vi "Quantum Composers 9000 Series Recall-Save Configuration.vi"() -> ()   [LabVIEW 2012]
doc: "This VI is an example of how to use subVIs from the QC 9000 series driver to programmatically recall/save a configuration from/to the unit's non-volatile memory.\n\n\nNotes:\n1) The pulse generator keypad is returned to \"Local\" mode when this VI terminates in order to restore manual control to the user.\n2) VISA Version 3.3 or higher must be installed to use this instrument driver."
uses:
  Support/Channel Parameters.ctl
  Support/System Parameters.ctl
  Quantum Composers 9000 Series.lvlib
panel:
  in  "Recall/Save (F:Read)":bool
  in  "Memory  (1)":i32=1
  in  "System Parameters":T1={"Sys Period"=0.1, "Sys Mode"=enum."Normal", "Sys Burst #"=10, "Sys DC On"=10, "Sys DC Off"=10, "Sys State"=TRUE, "Sys Gate"=TRUE, "Sys Trig Edge"=TRUE, "Sys Ext Mode"=enum."Disabled", "Sys Trig Lev"=2.5, "Sys Gate Lev "=2.5, "Sys Gate Mode"=enum."Disabled"} {"Sys Gate Lev" format="%.4p"; "Sys Trig Lev" format="%.4p"; "Sys Period" format="%.6p"}
  in  "VISA resource":refnum<visa-resource-name>="GPIB0::7::INSTR"
  in  "Channel Parameters":T2[](array[typedef]) {"Chan Sync Source" items=["System (To)", "Channel A", "Channel B", "Channel C", "Channel D", "Channel E", "Channel F", "Channel G", "Channel H"]; "Chan Width" format="%.3p"; "Chan Delay" format="%.3p"; "Chan Lev Adjust" format="%.3p"; "Channel" items=["Channel A"=1, "Channel B"=2, "Channel C"=3, "Channel D"=4, "Channel E"=5, "Channel F"=6, "Channel G"=7, "Channel H"=8]}
  # "9000 Series\nPulse Generator\nExample Program"
  # "Notes:\n1.  The channel parameters \"Burst #\", \"DC On\", \"DC Off\", and \"Adjustable\" are only updated when operating in the corresponding mode.\n2.  The system parameters  \"Burst #\", \"DC On\", \"DC Off\", and \"Trig Level\"` are only updated when operating in the corresponding mode."
  # "Input"
  # "Triggered"
  # "Gated"
  # "Mode"
  # "Burst"
  # "Duty\nCycle"
  # "Input"
  # "Normal\nSingle\nBurst"
  # "Burst"
  # "Duty Cycle"
  # "Output"
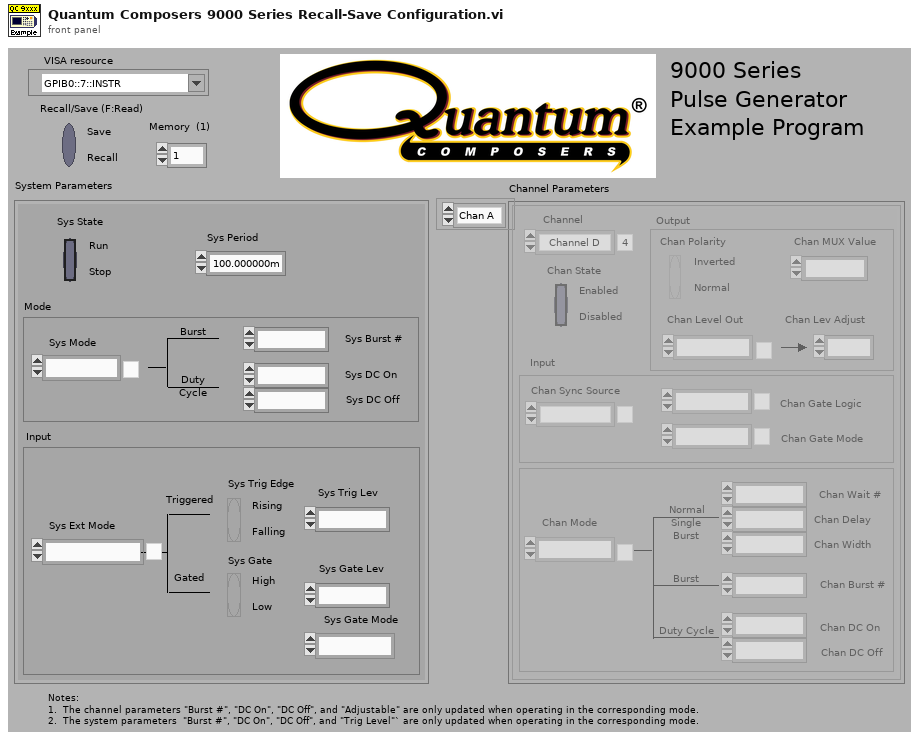
[diagram p1: front panel]
types:
  T1 = typedef "System Parameters.ctl" = cluster{"Sys Period":dbl, "Sys Mode":enum16{"Normal", "Single", "Burst", "Duty Cycle"}, "Sys Burst #":i32, "Sys DC On":i32, "Sys DC Off":i32, "Sys State":bool, "Sys Gate":bool, "Sys Trig Edge":bool, "Sys Ext Mode":enum16{"Disabled", "Triggered", "Gated", "Triggered & Gated"}, "Sys Trig Lev":dbl, "Sys Gate Lev ":dbl, "Sys Gate Mode":enum16{"Disabled", "Pulse Inhibit", "Output Inhibit", "Channel"}}
  T2 = typedef "Channel Parameters.ctl" = cluster{"Channel":i32, "Chan State":bool, "Chan Sync Source":i32, "Chan Gate Logic":enum16{"Disabled", "Low", "High"}, "Chan Mode":enum16{"Normal", "Single", "Burst", "Duty Cycle"}, "Chan Wait #":i32, "Chan Delay":dbl, "Chan Width":dbl, "Chan Burst #":i32, "Chan DC On":i32, "Chan DC Off":i32, "Chan Polarity":bool, "Chan MUX Value":i32, "Chan Level Out":enum16{"TTL", "Adjustable", "35 Volt", "Optical"}, "Chan Lev Adjust":dbl, "Chan Gate Mode":enum16{"Disabled", "Pulse Inhibit", "Output Inhibit"}}
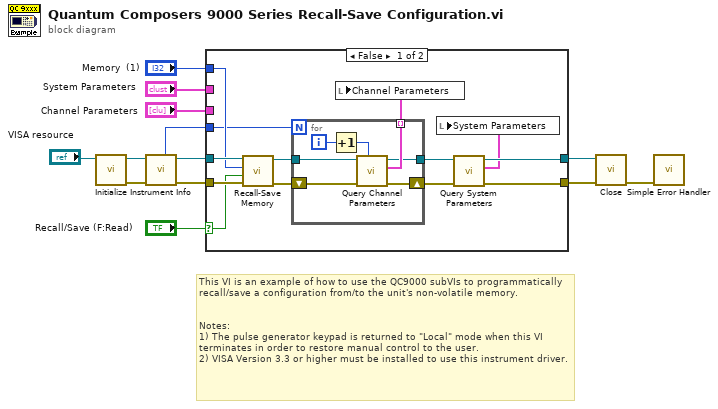
[diagram p0: block diagram]
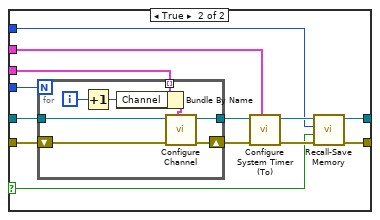
[diagram p2: hidden frame]
diagram:
  # "This VI is an example of how to use the QC9000 subVIs to programmatically recall/save a configuration from/to the unit's non-volatile memory.\n\n\nNotes:\n1) The pulse generator keypad is returned to \"Local\" mode when this VI terminates in order to restore manual control to the user.\n2) VISA Version 3.3 or higher must be installed to use this instrument driver."
  n1 = call "Initialize.vi"("VISA resource name"="VISA resource") -> ("error out"=w7:errorcluster, "VISA resource name out"=w6:refnum<visa-resource-name>)  [unwired: 9 in]
  n2 = call "Instrument Info.vi"("error in (no error)"=w7, "VISA resource name"=w6) -> ("error out"=w2:errorcluster, "VISA resource name out"=w3:refnum<visa-resource-name>, "Channels"=w5:i32)  [unwired: 6 in, 1 out]
  n3 = case shown="False" "Recall/Save (F:Read)" {
    selector: "Recall/Save (F:Read)" -> [w23 w34]
    tunnel: "Channel Parameters" -> [_ w46]
    tunnel: w3 -> [w26 w45]
    tunnel: w2 -> [w25 w44]
    tunnel: "System Parameters" -> [_ w43]
    tunnel: [w17 w38] -> w10
    tunnel: [w16 w37] -> w9
    tunnel: "Memory  (1)" -> [w24 w36]
    tunnel: w5 -> [w14 w35]
    frame False {
      n4 = call "Recall-Save Memory.vi"("error in (no error)"=w25, "Recall/Save (F:Read)"=w23, "Memory  (1)"=w24, "VISA resource name"=w26) -> ("error out"=w20:errorcluster, "VISA resource name out"=w22:refnum<visa-resource-name>)  [unwired: 6 in]
      n5 = for {
        N: w14 -> [_]
        tunnel: w22 -> [w33]
        tunnel: [w32] -> w21 mode=indexing
        shift-right: [w30] -> w18
        shift-left: w20 -> [w31]
        tunnel: [w29] -> w19
        i -> [w28]
        n6 = Increment(x=w28) -> (x+1=w27:i32)
        n7 = call "Query Channel Parameters.vi"("Channel (1:Chan A)"=w27, "error in (no error)"=w31, "VISA resource name"=w33) -> ("error out"=w30:errorcluster, "Chan Parameters"=w32:T2, "VISA resource name out"=w29:refnum<visa-resource-name>)  [unwired: 6 in]
      }
      n8 = local write "Channel Parameters"(w21) -> ()
      n9 = call "Query System Parameters.vi"("error in (no error)"=w18, "VISA resource name"=w19) -> ("error out"=w16:errorcluster, "System Parameters"=w15:T1, "VISA resource name out"=w17:refnum<visa-resource-name>)  [unwired: 7 in]
      n10 = local write "System Parameters"(w15) -> ()
    }
    frame True {
      n11 = for {
        N: w35 -> [_]
        tunnel: [w54] -> w42
        tunnel: w46 -> [w49] mode=indexing
        shift-right: [w53] -> w41
        shift-left: w44 -> [w52]
        tunnel: w45 -> [w51]
        i -> [w48]
        n12 = Increment(x=w48) -> (x+1=w47:i32)
        n13 = Bundle By Name(cluster=w49, "Channel"=w47) -> (w50:T2)
        n14 = call "Configure Channel.vi"("Chan Parameters"=w50, "error in (no error)"=w52, "VISA resource name"=w51) -> ("error out"=w53:errorcluster, "VISA resource name out"=w54:refnum<visa-resource-name>)  [unwired: 7 in]
      }
      n15 = call "Configure System Timer (To).vi"("System Parameters"=w43, "error in (no error)"=w41, "VISA resource name"=w42) -> ("error out"=w39:errorcluster, "VISA resource name out"=w40:refnum<visa-resource-name>)  [unwired: 7 in]
      n16 = call "Recall-Save Memory.vi"("error in (no error)"=w39, "Recall/Save (F:Read)"=w34, "Memory  (1)"=w36, "VISA resource name"=w40) -> ("error out"=w37:errorcluster, "VISA resource name out"=w38:refnum<visa-resource-name>)  [unwired: 6 in]
    }
  }
  n17 = call "Close.vi"("error in (no error)"=w9, "VISA resource name"=w10) -> ("error out"=w1:errorcluster)  [unwired: 9 in]
  n18 = call <vilib>:"Simple Error Handler.vi"("error in (no error)"=w1) -> ()  [unwired: 4 in, 5 out]
